vi "Configure Control AI Range(GS Scale).vi"(0 "VISA resource name":refnum<visa-resource-name>, 1 "Unit No. (0)":i32 min=0 max=6, 2 "Range, Span, Bias":T2={"GS Range (0 : 1-5V)"=0, "Enable Span (False)"=FALSE, "Lower Span (-2.0000)"=-2.0, "Upper Span (2.0000)"=2.0, "Bias (0)"=0.0} {"Upper Span (2.0000)" min=-99999.0 max=99999.0 step=1.0 format="%_5g"; "Lower Span (-2.0000)" min=-99999.0 max=99999.0 step=1.0 format="%_5g"; "GS Range (0 : 1-5V)" items=["1-5V", "0.4-2V"]}, 3 "Scaling":T1={"Floating point position (2)"=2, "Lower Scaling (0)"=0.0, "Upper Scaling (100.00)"=100.0, "Unit Character (\"\")"=""} {"Upper Scaling (100.00)" format="%_6g"; "Lower Scaling (0)" format="%_6g"; "Floating point position (2)" min=0 max=5 step=1}, 4 "Module No.(0)":i32 min=0 max=9, 5 "AI No.(1)":i32=1 min=1 max=2, 7 "error in (no error)":errorcluster) -> (20 "VISA resource name out":refnum<visa-resource-name>, 21 "AI No.":i32, 24 "Unit No.":i32, 25 "Module No.":i32, 27 "error out":errorcluster)   [LabVIEW 2020, in "Yokogawa GX Series.lvlib"]
doc: "Set GS Scale range of AI channel in PID module.\n\nCommand: SCtrlRangeAI"
uses:
  <instrlib>/Yokogawa GX Series/Yokogawa GX Series.lvlib
  <instrlib>/Yokogawa GX Series/Private/GS Range.vi
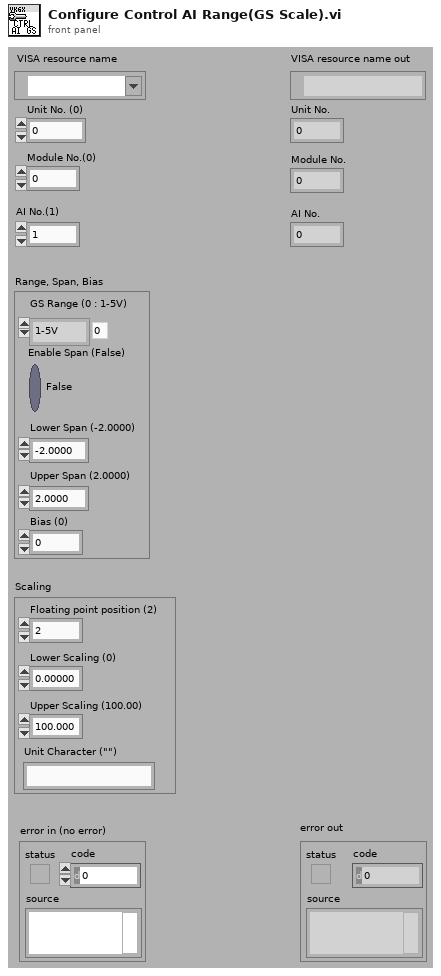
[diagram p1: front panel]
types:
  T1 = cluster{"Floating point position (2)":i32, "Lower Scaling (0)":dbl, "Upper Scaling (100.00)":dbl, "Unit Character (\"\")":string}
  T2 = cluster{"GS Range (0 : 1-5V)":i32, "Enable Span (False)":bool, "Lower Span (-2.0000)":dbl, "Upper Span (2.0000)":dbl, "Bias (0)":dbl}
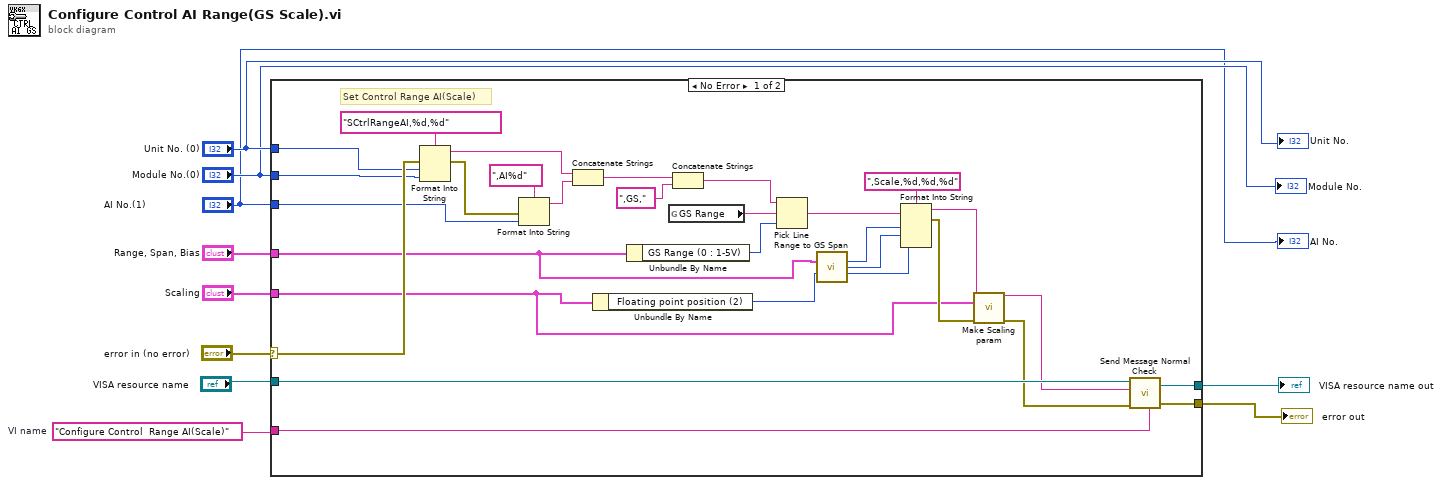
[diagram p0: block diagram]
diagram:
  w6 = "Configure Control  Range AI(Scale)"  # VI name
  n1 = case shown="No Error" "error in (no error)" {
    selector: "error in (no error)" -> [w36 w41]
    tunnel: [w40 w42] -> w10
    tunnel: [w39 w41] -> w9
    tunnel: "VISA resource name" -> [w38 w42]
    tunnel: w6 -> [w35 _]
    tunnel: "Unit No. (0)" -> [w34 _]
    tunnel: "Module No.(0)" -> [w33 _]
    tunnel: "AI No.(1)" -> [w31 _]
    tunnel: "Range, Span, Bias" -> [w14 _]
    tunnel: "Scaling" -> [w13 _]
    frame No Error {
      # "Set Control Range AI(Scale)"
      n2 = Format Into String(format string="SCtrlRangeAI,%d,%d", error in=w36, w34, w33) -> (resulting string=w29:string, error out=w30:errorcluster)  [unwired: 1 in]
      n3 = Format Into String(format string=",AI%d", error in=w30, w31) -> (resulting string=w28:string)  [unwired: 1 in, 1 out]
      n4 = Concatenate Strings(w29, w28) -> (w23:string)
      n5 = Unbundle By Name(w13) -> ("Floating point position (2)"=w15:i32)
      n6 = Unbundle By Name(w14) -> ("GS Range (0 : 1-5V)"=w26:i32)
      n7 = global read "GS Range.vi" "GS Range"() -> (w24:string)
      n8 = Concatenate Strings(w23, ",GS,") -> (w27:string)
      n9 = Pick Line(string ("")=w27, multi-line string=w24, line index=w26) -> (output string=w16:string)
      n10 = call <instrlib>:"Range to GS Span.vi"("Range and span"=w14, "Floating Point Position (2)"=w15) -> ("Lower Span"=w21:i32, "Upper Span"=w20:i32, "Bias"=w19:i32)  [unwired: 11 in]
      n11 = Format Into String(format string=",Scale,%d,%d,%d", initial string=w16, w21, w20, w19) -> (resulting string=w18:string, error out=w17:errorcluster)  [unwired: 1 in]
      n12 = call <instrlib>:"Make Scaling param.vi"("String (\"\")"=w18, "Scaling"=w13, "error in (no error)"=w17) -> ("String After"=w12:string, "error out"=w11:errorcluster)  [unwired: 11 in]
      n13 = call <instrlib>:"Send Message Normal Check.vi"("Source (\"\")"=w35, "error in (no error)"=w11, "Send Message (\"\")"=w12, "VISA resource name"=w38) -> ("error out"=w39:errorcluster, "VISA resource name out"=w40:refnum<visa-resource-name>)  [unwired: 2 in, 4 out]
    }
    frame Error {
    }
  }
  "error out" <- w9
  "VISA resource name out" <- w10
  "Unit No." <- "Unit No. (0)"
  "Module No." <- "Module No.(0)"
  "AI No." <- "AI No.(1)"
